vi "find_FrontPanel_Ref.vi"(8 "error in (no error)":errorcluster, 10 "FrontPanelObject name":string(combo), 11 "Ref_RunScriptWindow":refnum<vi>) -> (0 "error out":errorcluster, 2 "FrontPanelObject ref out":refnum<vi>, 3 "Ref_RunScriptWindow out":refnum<vi>)   [LabVIEW 2018]
doc: "finds the reference of the desired FrontPanelObject"
panel:
  out "Array":string[](array[string])
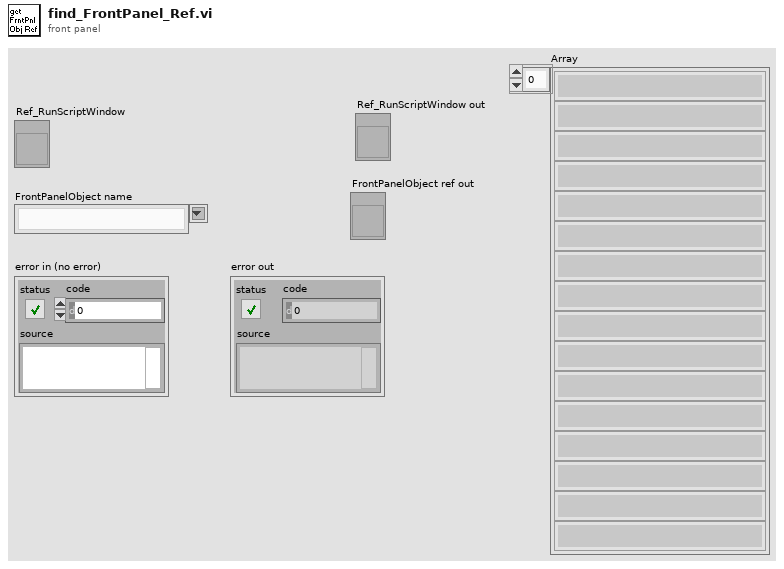
[diagram p1: front panel]
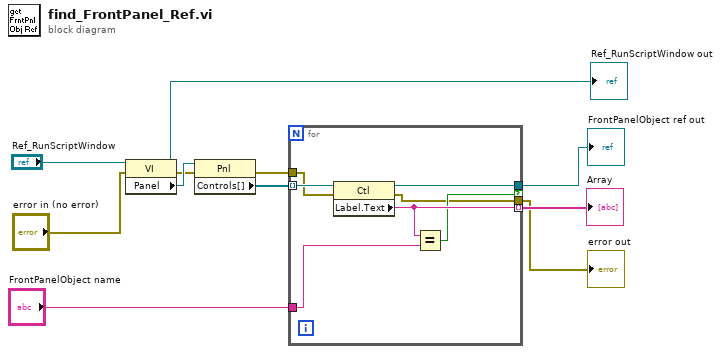
[diagram p0: block diagram]
diagram:
  n1 = property class="VI"(reference="Ref_RunScriptWindow", error in="error in (no error)") -> (reference out=→"Ref_RunScriptWindow out":refnum<vi>, error out=w9:errorcluster, "Panel"=w10:refnum<vi>)
  n2 = property class="Pnl"(reference=w10, error in=w9) -> (error out=w6:errorcluster, "Controls[]"=w4:refnum<vi>[])  [unwired: 1 out]
  n3 = for {
    tunnel: w4 -> [w18] mode=indexing
    tunnel: [w16] -> w8 mode=indexing
    tunnel: w6 -> [w13]
    tunnel: "FrontPanelObject name" -> [w17]
    tunnel: [w14] -> w3 if=w15
    tunnel: [w12] -> w2
    n4 = property class="Ctl"(reference=w18, error in=w13) -> (reference out=w14:refnum<vi>, error out=w12:errorcluster, "Label.Text"=w16:string)
    n5 = Equal?(x=w16, y=w17) -> (x = y?=w15:bool)
  }
  "Array" <- w8
  "error out" <- w2
  "FrontPanelObject ref out" <- w3
